vi "Bool.vi"(4 "Array":bool[](array[boolean])) -> (1 "Abs_Boolean_1D.lvclass":refnum<class "Abs_Boolean_1D.lvclass">)   [LabVIEW 2021, in "Const_Bool_1D.lvclass"]
uses:
  Const_Bool_1D.lvclass
  Const_Bool_1D.lvclass/Const_Bool_1D.ctl
  C:/TSA/LV_Abstract/Source/Abs_Types/Boolean_1D/Abs_Boolean_1D.lvclass
  C:/TSA/LV_Abstract/Source/Abs_Types/Value/Abs_Value.lvclass
  C:/TSA/LV_Abstract/Source/Abs_Types/Type/Abs_Type.lvclass
  C:/TSA/LV_Abstract/Source/Abs_Types/Interfaces/Array1D/Array1D.lvclass
  C:/TSA/LV_Abstract/Source/Abs_Types/Interfaces/Array1D_Bool/Array1D_Bool.lvclass
  C:/TSA/LV_Abstract/Source/Constants/Support/Bool_1D/Const_Bool_1D.lvclass
  C:/TSA/LV_Abstract/Source/Constants/Support/Interface/Const_Intf.lvclass
  Abs_Types/Boolean_1D/Abs_Boolean_1D.lvclass
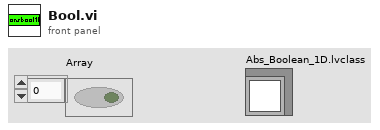
[diagram p1: front panel]
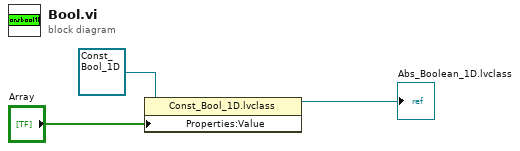
[diagram p0: block diagram]
diagram:
  n1 = property class="Const_Bool_1D.lvclass"(reference=refnum<class "Const_Bool_1D.lvclass"> refnum ("Constants.lvlib:Boolean.lvclass"), "Properties:Value"="Array") -> (reference out=→"Abs_Boolean_1D.lvclass":refnum<class "Const_Bool_1D.lvclass">)  [unwired: 1 in, 1 out]
